vi "Send DAQ Data Along Notifier.vi"(0 "Notifier Name":string, 1 "Experimental Data":dbl[][](array[numeric])) -> ()   [LabVIEW 2013]
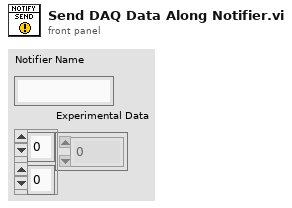
[diagram p1: front panel]
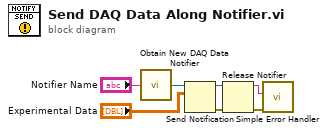
[diagram p0: block diagram]
diagram:
  n1 = call "Obtain New DAQ Data Notifier.vi"("Notifier Name"="Notifier Name") -> ("DAQ Data Notifier"=w5:refnum<notifier>)
  n2 = Send Notification(notification="Experimental Data", notifier=w5) -> (notifier out=w6:refnum<notifier>, error out=w2:errorcluster)  [unwired: 1 in]
  n3 = Release Notifier(notifier=w6, error in (no error)=w2) -> (notifier name=w7:string, error out=w1:errorcluster)  [unwired: 1 in, 1 out]
  n4 = call <vilib>:"Simple Error Handler.vi"("error source (\" \")"=w7, "error in (no error)"=w1) -> ()  [unwired: 3 in, 5 out]
